vi "RegisterCallback.vi"(8 "error in (no error)":errorcluster, 11 "subscriber in":refnum<class "IcmMessageSubscriber.lvclass">) -> (0 "error out":errorcluster, 2 "callback":refnum<user-event>, 3 "subscriber out":refnum<class "IcmMessageSubscriber.lvclass">)   [LabVIEW 2017, in "IcmMessageSubscriber.lvclass"]
doc: "Registers a callback to the message bus that causes the bus to return messages to the service."
uses:
  <vilib>/addons/InsightCM/MessageBus/MessageSubscriber/IcmMessageSubscriber.lvclass
  <vilib>/addons/InsightCM/MessageBus/Base/controls/MessageWrapper.ctl
  <vilib>/addons/InsightCM/MessageBus/Base/controls/Message.ctl
  <vilib>/addons/InsightCM/MessageBus/Base/controls/MessageHeader.ctl
  <vilib>/addons/InsightCM/MessageBus/Base/controls/KeyValuePair.ctl
  <vilib>/addons/InsightCM/MessageBus/MessageSubscriber/IcmMessageSubscriber.lvclass/IcmMessageSubscriber.ctl
  C:/Program Files (x86)/National Instruments/LabVIEW 2017/vi.lib/addons/InsightCM/Binaries/LabviewMessageAdapter.dll
  Binaries/LabviewMessageAdapter.dll
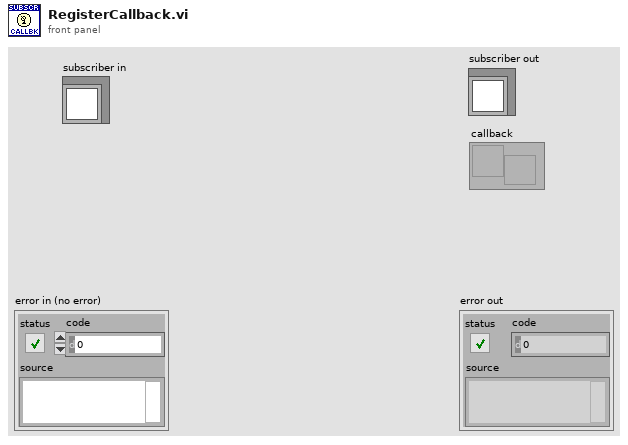
[diagram p1: front panel]
types:
  T1 = typedef "MessageWrapper.ctl" = cluster{"Message":T2}
  T2 = typedef "Message.ctl" = cluster{"Header":T3, "Body":u8[]}
  T3 = typedef "MessageHeader.ctl" = cluster{"MessageName":string, "Timestamp":i64, "CorrelationId":string, "ContentType":string, "RoutingKey":string, "Properties":T4[]}
  T4 = typedef "KeyValuePair.ctl" = cluster{"Key":string, "Value":string}
  T5 = typedef "MessageSubscriberDvr.ctl" = refnum<data-value>
  T6 = typedef "MessageSubscriberData.ctl" = cluster{"Subscriber":refnum<k24>}
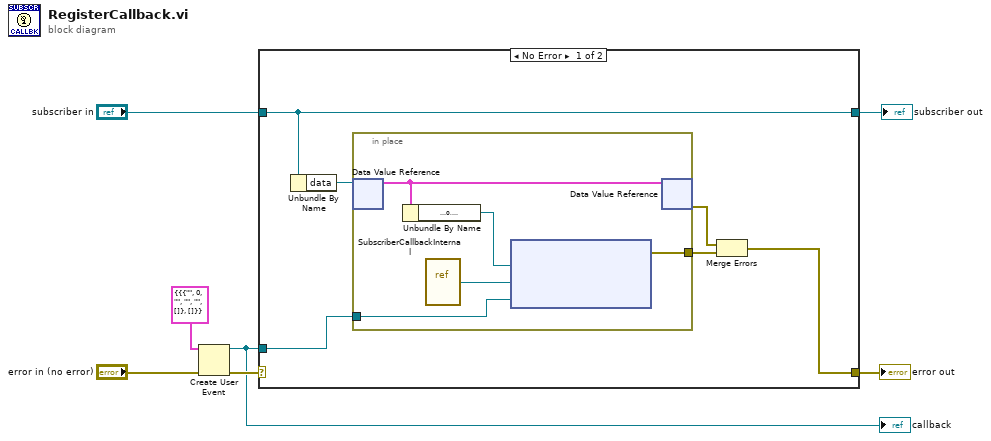
[diagram p0: block diagram]
diagram:
  n1 = Create User Event(user event datatype=T1 {"Message"={"Header"={"MessageName"="", "Timestamp"=0, "CorrelationId"="", "ContentType"="", "RoutingKey"="", "Properties"=[]}, "Body"=[]}} ("Message"), error in="error in (no error)") -> (user event=w4:refnum<user-event>, error out=w5:errorcluster)
  "callback" <- w4
  n2 = case shown="No Error" w5 {
    selector: w5 -> [_ w20]
    tunnel: [w9 w20] -> w7
    tunnel: w4 -> [w12 _]
    tunnel: "subscriber in" -> [w8 w19]
    tunnel: [w8 w19] -> w2
    frame No Error {
      n3 = Unbundle By Name(w8) -> ("data"=w13:T5)
      n4 = in-place {
        in-place-border: w12 -> [w15]
        in-place-border: [w14] -> w10
        n5 = in-place-dvr #1(w13) -> (w17:T6)  [unwired: 1 out]
        n6 = Unbundle By Name(w17) -> ("Subscriber"=w18:refnum<k24>)
        n7 = vi-ref <vilib>:"SubscriberCallbackInternal.vi"() -> ("vi reference"=w16:refnum<vi>)
        n8 = node(w18, w16, w15) -> (w14:errorcluster)  [unwired: 2 in, 1 out]
        n9 = in-place-dvr #1(w17) -> (w11:errorcluster)  [unwired: 1 out]
      }
      n10 = Merge Errors(w11, w10) -> (w9:errorcluster)
    }
    frame Error {
    }
  }
  "error out" <- w7
  "subscriber out" <- w2
